vi "DockerTools - Remove container by ID.vi"(8 "error in":errorcluster, 11 "String":string) -> (0 "error out":errorcluster)   [LabVIEW 2017]
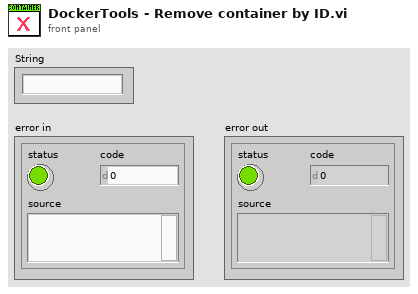
[diagram p1: front panel]
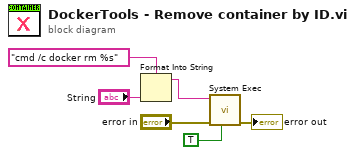
[diagram p0: block diagram]
diagram:
  n1 = Format Into String(format string="cmd /c docker rm %s" ("command line"), "String") -> (resulting string=w3:string)  [unwired: 2 in, 1 out]
  n2 = call <vilib>:"System Exec.vi"("run minimized? (F)"=TRUE, "error in (no error)"="error in", "command line"=w3) -> ("error out"=→"error out":errorcluster)  [unwired: 5 in, 3 out]
